vi "Channel Interface.vi"(8 "error in (no error)":errorcluster, 11 "Node Ptr":T1 format="%.0x") -> (0 "error out":errorcluster)   [LabVIEW 2017, in "SLSC EDS System Explorer.lvlib"]
uses:
  SLSC EDS System Explorer.lvlib
  <vilib>/NI Veristand/Custom Device API/Custom Device Item Ref.ctl
  <vilib>/NI Veristand/Custom Device API/Custom Device Channel Type.ctl
  <vilib>/NI Veristand/Custom Device Tools/Custom Device Utility Library/Search Direction.ctl
  <vilib>/Utility/miscctls.llb/LVStringsAndValuesArrayTypeDef_U16.ctl
  Shared/Constants.vi
  <vilib>/NI Veristand/Custom Device API/Get Item Property (String).vi
  <vilib>/NI Veristand/Custom Device Tools/Custom Device Utility Library/NI VeriStand - Search for Item by GUID.vi
  <vilib>/NI VeriStand/Custom Device API/Custom Device API.lvlib
  Shared/SLSC EDS Shared.lvlib
  <vilib>/NI VeriStand/Custom Device Tools/Custom Device Utility Library/Custom Device Utility Library.lvlib
  SLSC CD API/SLSC CD Shared/SLSC CD Shared.lvlib
  <vilib>/NI Veristand/Custom Device Tools/Custom Device Utility Library/NI VeriStand - Search for Item by Name.vi
  SLSC UI API/SLSC Tree Control.lvlib
  SLSC CD API/SLSC CD System Explorer/SLSC CD System Explorer.lvlib
panel:
  in  "Property tree":string[](tree)
  out "Physical Channel":string
  out "Property/Command Name":string
  out "Datatype":string
  in  "U8":u8 format="%.0x"
  in  "I8":i8
  in  "U32":u32 format="%.0x"
  in  "I32":i32
  in  "U64":u64 format="%.0x"
  in  "I64":i64
  in  "Ring":u16(ring)
  in  "DBL":dbl format="%#_16g"
  out "Documentation":string
  in  "Default Value":dbl
  out "Access":i32(ring) items=["None", "Read Only", "Write Only", "Read/Write"]
  out "SLSC Debugging Information":string
  in  "Header":cluster{"Section Name":string}={"Section Name"="Custom Device Item Settings"}
  out "Description":string
  out "Name":string
  # "Default Value"
  # "Channel Value"
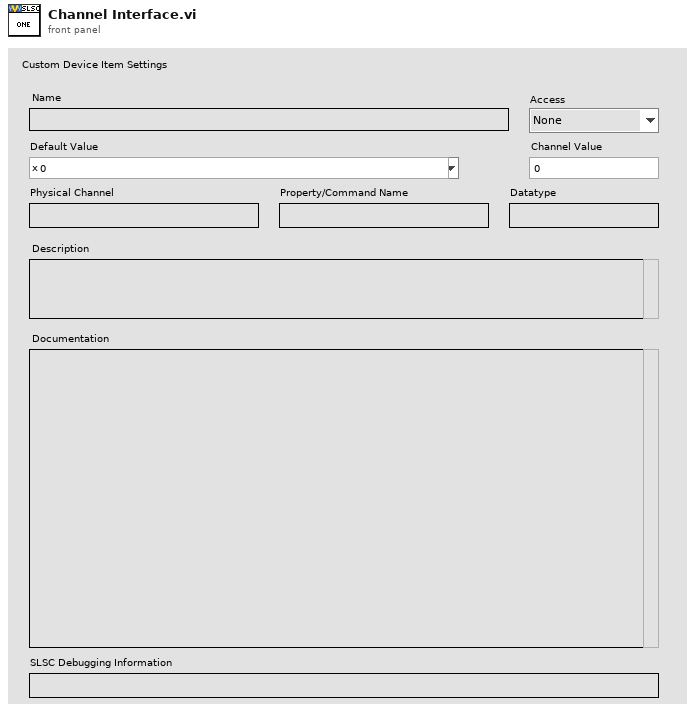
[diagram p1: front panel]
types:
  T1 = typedef "Custom Device API.lvlib/Custom Device Item Ref.ctl" = u64
  T2 = enum8{"Enabled", "Disabled", "Disabled and Grayed Out"}
  T3 = typedef "Custom Device Utility Library.lvlib/Search Direction.ctl" = enum16{"Down", "Up"}
  T4 = typedef "Custom Device API.lvlib/Custom Device Channel Type.ctl" = enum16{"Input", "Output"}
  T5 = typedef "LVStringsAndValuesArrayTypeDef_U16.ctl" = cluster{"String":string, "Value":u16}[]
  T6 = typedef "Custom Device API.lvlib/Custom Device Item Info.ctl" = cluster{"Name":string, "Is Channel":bool, "GUID":string, "Is Waveform":bool}
  T7 = typedef "EDSjsonStructure.ctl" = cluster{"vendorNum":u32, "vendorName":string, "vendorPrefix":string, "productNum":u32, "productName":string, "capsVersion":string, "capsSpecVersion":u32, "capsSpecOldestCompatibleVersion":u32, "enums":T8[], "properties":T9[], "commands":T10[], "scales":T11[], "physicalChannels":T12[], "registerMap":cluster{"registers":T13[]}}
  T8 = typedef "enum.ctl" = cluster{"name":string, "description-en":string, "values":cluster{"name":string, "description-en":string, "value":i32}[]}
  T9 = typedef "property.ctl" = cluster{"name":string, "description-en":string, "documentation-en":string, "dataType":string, "bitfield":string, "access":string, "scale":string, "value":variant, "min":variant, "max":variant, "default value":variant}
  T10 = typedef "command.ctl" = cluster{"name":string, "description-en":string, "documentation-en":string, "startBitfield":string, "waitTimeInMs":i32, "doneBitfield":string, "doneInterrupt":string, "doneTimeoutInMs":i32, "value":variant}
  T11 = typedef "scale.ctl" = cluster{"name":string, "description-en":string, "m":dbl, "b":dbl, "forwardCoeffs":dbl[], "reverseCoeffs":dbl[], "coercion":string, "table":cluster{"scaled":dbl, "unscaled":dbl}[]}
  T12 = typedef "physicalChannel.ctl" = cluster{"name":string, "description-en":string, "commands":T10[], "properties":T9[]}
  T13 = typedef "register.ctl" = cluster{"name":string, "description-en":string, "access":string, "address":u32, "size":u32, "bitfields":cluster{"name":string, "description-en":string, "offset":u32, "size":u32, "signed":bool, "strobe":bool}[]}
  T14 = typedef "Custom Device API.lvlib/Custom Device Channel.ctl" = cluster{"Type":T4, "Units":string, "Default Value":dbl, "Faultable":bool, "Scalable":bool}
  T15 = cluster{"Left Cell String":string, "Child Text":string[], "Child Tag":string, "Item Indent":i32, "Child Only?":bool, "Glyph Index":i32}[]
  T16 = cluster{"Left Cell String":string, "Child Text":string[], "Child Tag":string, "Item Indent":i32, "Child Only?":bool, "Glyph Index":i32}
  T17 = cluster{"name":string, "description-en":string, "value":i32}[]
  T18 = typedef "Custom Device API.lvlib/Custom Device Commands.ctl" = enum16{"Default", "Item renamed", "Shutdown", "Dynamic button pressed"}
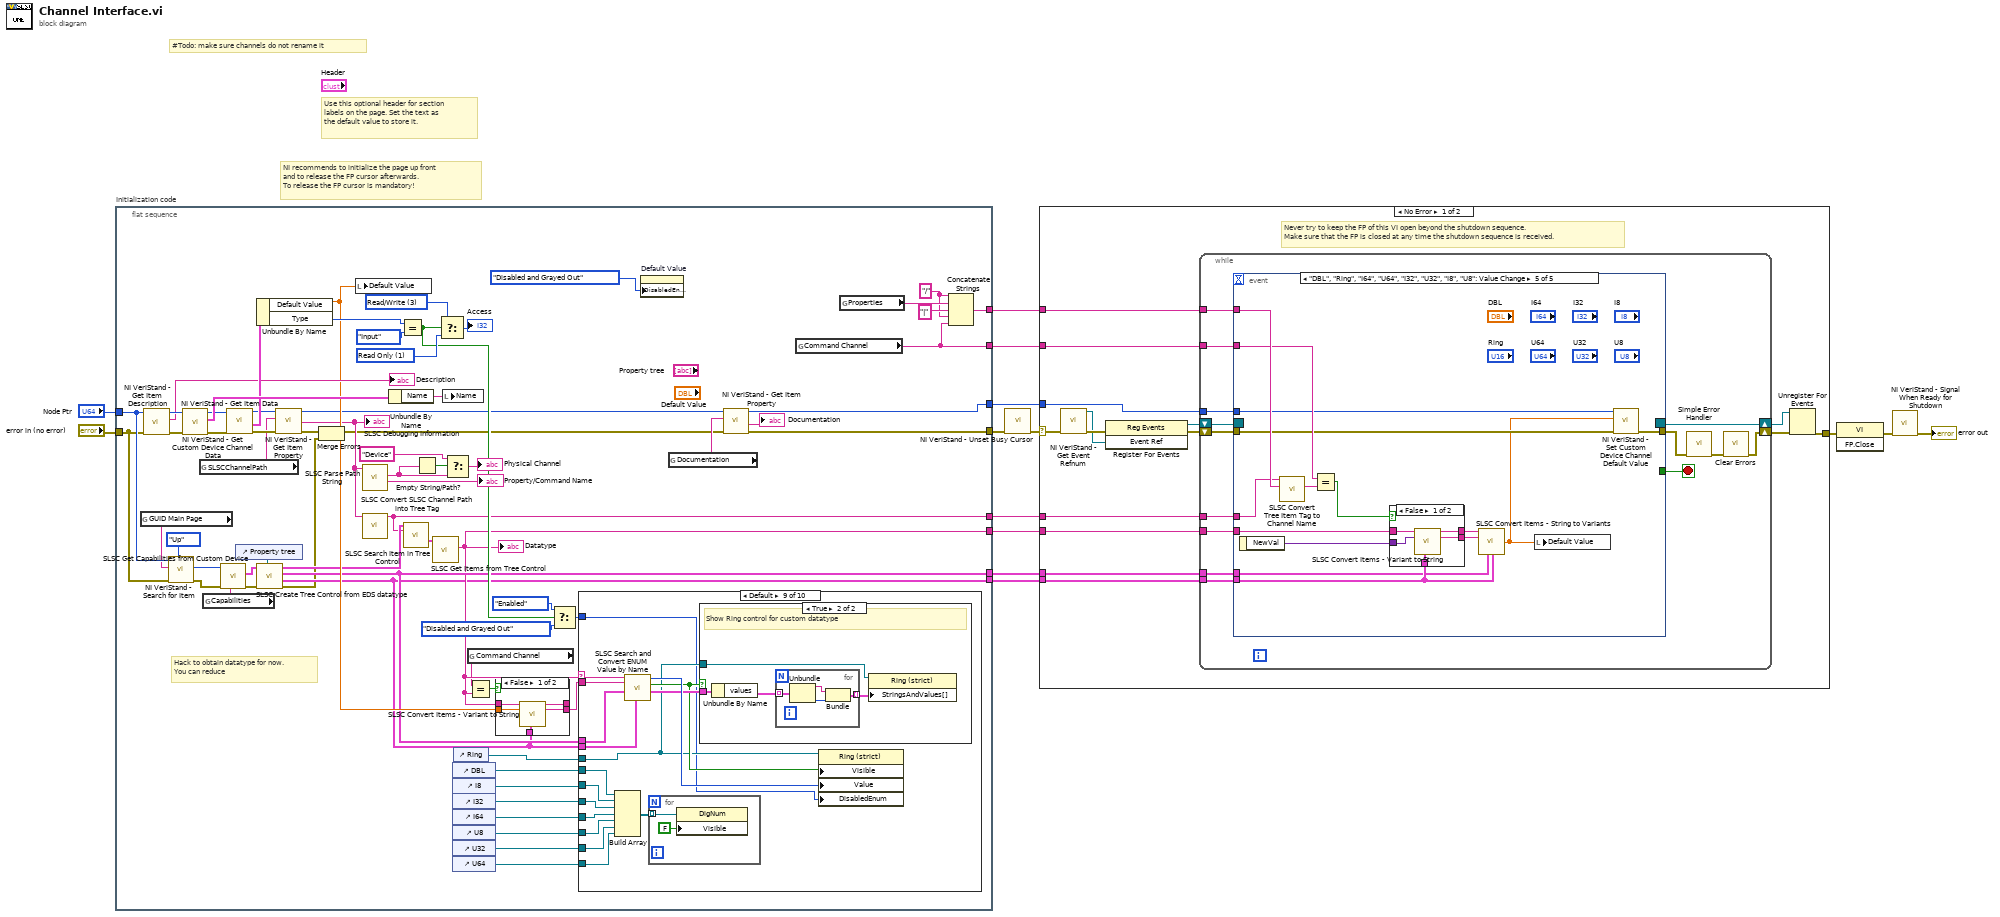
[diagram p0: block diagram]
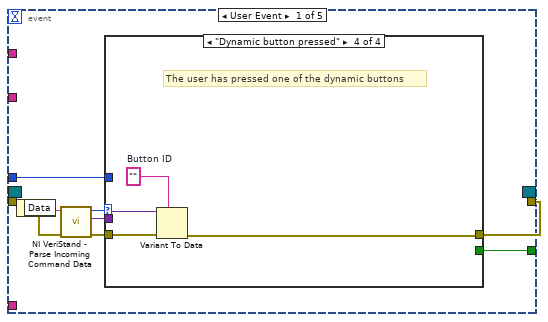
[diagram p2: hidden frame]
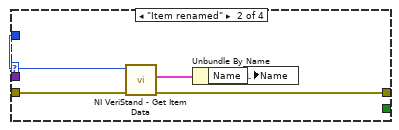
[diagram p4: hidden frame]
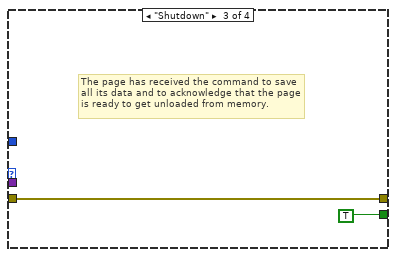
[diagram p5: hidden frame]
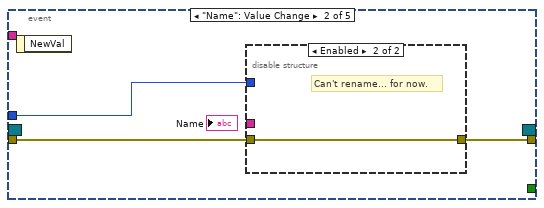
[diagram p6: hidden frame]
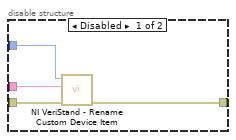
[diagram p7: hidden frame]
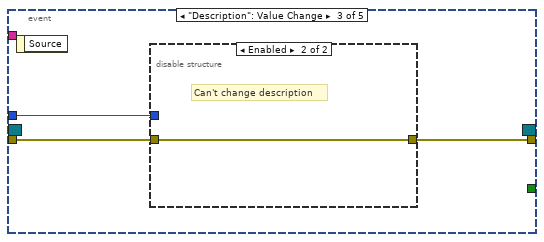
[diagram p8: hidden frame]
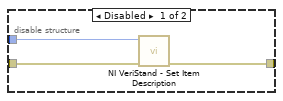
[diagram p9: hidden frame]
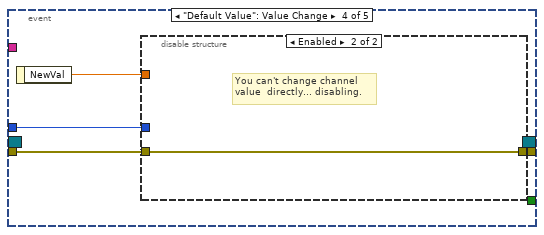
[diagram p10: hidden frame]
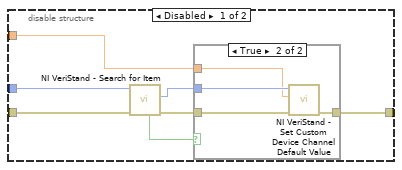
[diagram p11: hidden frame]
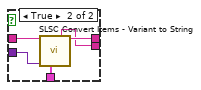
[diagram p13: hidden frame]
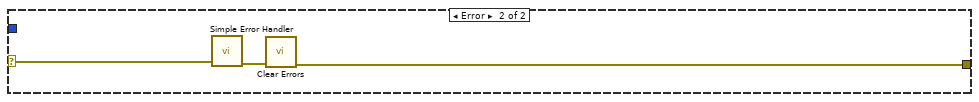
[diagram p14: hidden frame]
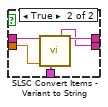
[diagram p15: hidden frame]
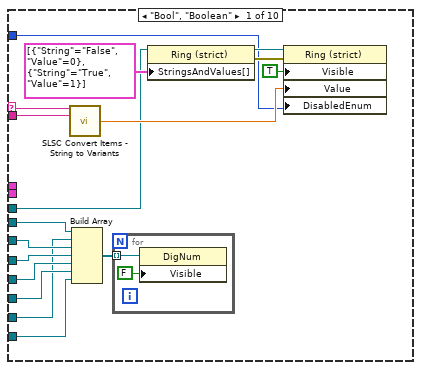
[diagram p16: hidden frame]
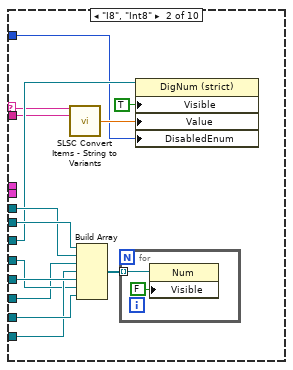
[diagram p17: hidden frame]
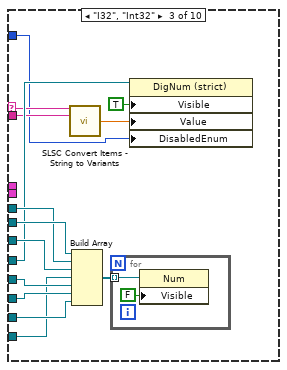
[diagram p18: hidden frame]
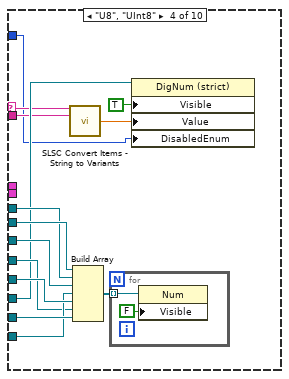
[diagram p19: hidden frame]
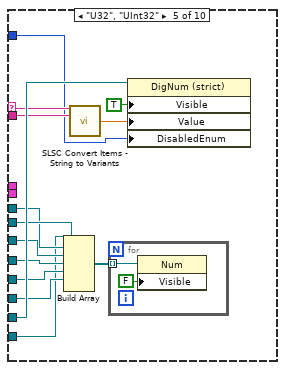
[diagram p20: hidden frame]
diagram:
  # "#Todo: make sure channels do not rename it"
  # "Use this optional header for section labels on the page. Set the text as the default value to store it."
  # "NI recommends to initialize the page up front\nand to release the FP cursor afterwards.\nTo release the FP cursor is mandatory!"
  n1 = flat-sequence "Initialization code" {
    tunnel: "error in (no error)" -> [w28]
    tunnel: "Node Ptr" -> [w53]
    tunnel: [w66] -> w10
    tunnel: [w23] -> w7
    tunnel: [w58] -> w6
    tunnel: [w49] -> w5
    tunnel: [w30] -> w4
    tunnel: [w36] -> w3
    tunnel: [w31] -> w2
    tunnel: [w32] -> w1
    frame #0 {
      w59 = "/" ("string")
      w79 = 1 items=["None", "Read Only", "Write Only", "Read/Write"] ("Access")
      w78 = 3 items=["None", "Read Only", "Write Only", "Read/Write"] ("Access")
      # "Hack to obtain datatype for now.\nYou can reduce"
      n2 = global read "Constants.vi" "GUID Main Page"() -> (w52:string)
      n3 = call <vilib>:"NI VeriStand - Get Item Description.vi"("error in (no error)"=w28, "Item Ref in"=w53) -> ("error out"=w81:errorcluster, "Description"=→"Description":string, "Item Ref out"=w82:T1)  [unwired: 7 out]
      n4 = call-poly <vilib>:"NI VeriStand - Search for Item.vi"("Direction (Down)"=Search_Direction."Up", "error in"=w28, "Item GUID"=w52, "Section Ref in"=w53) -> ("error out"=w29:errorcluster, "Item Ref"=w54:T1)  [unwired: 4 in, 2 out]
      n5 = call <vilib>:"NI VeriStand - Get Item Data.vi"("error in (no error)"=w81, "Item Ref in"=w82) -> ("error out"=w71:errorcluster, "Item Info"=w80:T6, "Item Ref out"=w72:T1)  [unwired: 7 out]
      n6 = global read "Constants.vi" "SLSCChannelPath"() -> (w70:string)
      n7 = global read "Constants.vi" "Capabilities"() -> (w62:string)
      n8 = call "SLSC Get Capabilities from Custom Device.vi"("Property Name"=w62, "error in (no error)"=w29, "Device Item Ref in"=w54) -> ("error out"=w25:errorcluster, "data"=w37:T7)  [unwired: 3 in, 4 out]
      n9 = call <vilib>:"NI VeriStand - Get Custom Device Channel Data.vi"("error in (no error)"=w71, "Channel Ref in"=w72) -> ("error out"=w74:errorcluster, "Channel"=w73:T14, "Channel Ref out"=w68:T1)  [unwired: 4 in, 3 out]
      n10 = control-ref of="Property tree"() -> (w38:refnum<vi>)
      n11 = Unbundle By Name(w73) -> ("Default Value"=w50:dbl, "Type"=w75:T4)
      n12 = call "SLSC Create Tree Control from EDS datatype.vi"("Property Tree"=w38, "error in (no error)"=w25, "SLSC EDS module"=w37) -> ("error out"=w19:errorcluster, "Enum Strings"=w30:cluster{"name":string, string}[], "Enums"=w36:T8[], "SLSC Output Tree"=w35:T15)  [unwired: 5 in]
      n13 = call-poly <vilib>:"NI VeriStand - Get Item Property.vi"("error in (no error)"=w74, "Property Name"=w70, "Item Ref in"=w68) -> ("error out"=w21:errorcluster, "Value"=w34:string, "Item Ref out"=w22:T1)  [unwired: 5 in, 1 out]
      "SLSC Debugging Information" <- w34
      n14 = Merge Errors(w21, w19) -> (w20:errorcluster)
      n15 = local write "Default Value"(w50) -> ()
      n16 = call "SLSC Parse Path String.vi"("SLSC Channel Path"=w34) -> ("Property or Command"=→"Property/Command Name":string, "Physical Channel"=w40:string)  [unwired: 7 in, 2 out]
      n17 = call "SLSC Convert SLSC Channel Path into Tree Tag.vi"("SLSC Channel Path"=w34) -> ("Tree Item Channel"=w32:string)  [unwired: 9 in, 1 out]
      n18 = Unbundle By Name(w80) -> ("Name"=w63:string)
      n19 = Equal?(x=w75, y=Custom_Device_Channel_Type."Input") -> (x = y?=w64:bool)
      n20 = call "SLSC Search Item in Tree Control.vi"("SLSC Output Tree"=w35, "Item Tag"=w32) -> ("Item"=w33:T16)  [unwired: 10 in, 3 out]
      n21 = Empty String/Path?(string/path=w40) -> (empty?=w42:bool)
      n22 = call "SLSC Get Items from Tree Control.vi"("Item"=w33) -> ("Datatype"=w31:string)  [unwired: 6 in, 4 out]
      "Datatype" <- w31
      n23 = Select(t=w78, s=w64, f=w79) -> (s? t:f=→"Access":i32)
      n24 = local write "Name"(w63) -> ()
      n25 = Select(t="Device", s=w42, f=w40) -> (s? t:f=→"Physical Channel":string)
      n26 = control-ref of="DBL"() -> (w44:refnum<vi>)
      n27 = control-ref of="I8"() -> (w57:refnum<vi>)
      n28 = control-ref of="I32"() -> (w56:refnum<vi>)
      n29 = control-ref of="I64"() -> (w45:refnum<vi>)
      n30 = control-ref of="U8"() -> (w48:refnum<vi>)
      n31 = control-ref of="U32"() -> (w47:refnum<vi>)
      n32 = control-ref of="U64"() -> (w46:refnum<vi>)
      n33 = control-ref of="Ring"() -> (w16:refnum<vi>)
      n34 = global read "Constants.vi" "Command Channel"() -> (w24:string)
      n35 = Equal?(x=w24, y=w31) -> (x = y?=w27:bool)
      n36 = case shown="False" w27 {
        tunnel: w50 -> [w87 w89]
        tunnel: [w86 w88] -> w26
        tunnel: [w85 w92] -> _
        tunnel: w31 -> [w84 w91]
        tunnel: w30 -> [w83 w90]
        frame False {
          n37 = call "SLSC Convert Items - Variant to String.vi"("Datatype"=w84, "value"=w87, "Enum string"=w83) -> ("Output data type"=w85:string, "string data value"=w86:string)  [unwired: 6 in, 5 out]
        }
        frame True {
          n38 = call "SLSC Convert Items - Variant to String.vi"("Datatype"=w91, "reset value"=w89, "Enum string"=w90) -> ("string data reset value"=w88:string, "Output data type"=w92:string)  [unwired: 6 in, 5 out]
        }
      }
      n39 = Select(t=T2."Enabled" ("Disabled"), s=w64, f=T2."Disabled and Grayed Out" ("Disabled")) -> (s? t:f=w15:T2)
      n40 = case shown="Default" w31 {
        selector: w31 -> [w99 w116 w132 w148 w164 w178 w198 w216 w233 w264]
        tunnel: w16 -> [w95 w124 w140 w156 w171 w190 w208 w225 w229 w256]
        tunnel: w47 -> [w102 w121 w135 w152 w173 w185 w202 w219 w238 w268]
        tunnel: w44 -> [w109 w125 w141 w157 w172 w191 w209 w218 w243 w273]
        tunnel: w57 -> [w108 w117 w139 w155 w170 w189 w207 w224 w242 w272]
        tunnel: w56 -> [w107 w119 w133 w150 w169 w188 w206 w223 w241 w271]
        tunnel: w45 -> [w106 w123 w138 w154 w168 w183 w205 w222 w240 w270]
        tunnel: w48 -> [w105 w118 w137 w149 w167 w187 w204 w221 w239 w269]
        tunnel: w46 -> [w104 w120 w134 w151 w166 w184 w201 w217 w237 w267]
        tunnel: w36 -> [_ _ _ _ _ _ _ _ w244 _]
        tunnel: w26 -> [w98 w115 w131 w147 w163 w177 w197 w215 w235 w265]
        tunnel: w30 -> [_ _ _ _ _ _ _ _ w234 _]
        tunnel: w15 -> [w93 w112 w128 w144 w160 w176 w194 w212 w228 _]
        frame "Bool", "Boolean" {
          n41 = call "SLSC Convert Items - String to Variants.vi"("Datatype"=w99, "Value"=w98) -> ("Value (DBL)"=w97:dbl)  [unwired: 10 in, 3 out]
          n42 = Build Array(w109, w102, w108, w107, w106, w105, w104) -> (w103:refnum<vi>[])
          n43 = for {
            tunnel: w103 -> [w111] mode=indexing
            n44 = property class="DigNum"(reference=w111, "Visible"=FALSE) -> ()  [unwired: 1 in, 2 out]
          }
          n45 = property on="Property Node" class="Ring (strict)"(reference=w95, "StringsAndValues[]"=T5 [{"String"="False", "Value"=0}, {"String"="True", "Value"=1}] ("Strings And Values []")) -> (reference out=w94:refnum<vi>, error out=w100:errorcluster)  [unwired: 1 in]
          n46 = property class="Ring (strict)"(reference=w94, error in=w100, "Visible"=TRUE, "Value"=w97, "DisabledEnum"=w93) -> ()  [unwired: 2 out]
        }
        frame "I8", "Int8" {
          n47 = call "SLSC Convert Items - String to Variants.vi"("Datatype"=w116, "Value"=w115) -> ("Value (DBL)"=w114:dbl)  [unwired: 10 in, 3 out]
          n48 = Build Array(w125, w124, w118, w120, w123, w119, w121) -> (w122:refnum<vi>[])
          n49 = for {
            tunnel: w122 -> [w127] mode=indexing
            n50 = property class="Num"(reference=w127, "Visible"=FALSE) -> ()  [unwired: 1 in, 2 out]
          }
          n51 = property class="DigNum (strict)"(reference=w117, "Visible"=TRUE, "Value"=w114, "DisabledEnum"=w112) -> ()  [unwired: 1 in, 2 out]
        }
        frame "I32", "Int32" {
          n52 = call "SLSC Convert Items - String to Variants.vi"("Datatype"=w132, "Value"=w131) -> ("Value (DBL)"=w130:dbl)  [unwired: 10 in, 3 out]
          n53 = Build Array(w141, w140, w139, w134, w138, w137, w135) -> (w136:refnum<vi>[])
          n54 = for {
            tunnel: w136 -> [w143] mode=indexing
            n55 = property class="Num"(reference=w143, "Visible"=FALSE) -> ()  [unwired: 1 in, 2 out]
          }
          n56 = property class="DigNum (strict)"(reference=w133, "Visible"=TRUE, "Value"=w130, "DisabledEnum"=w128) -> ()  [unwired: 1 in, 2 out]
        }
        frame "U8", "UInt8" {
          n57 = call "SLSC Convert Items - String to Variants.vi"("Datatype"=w148, "Value"=w147) -> ("Value (DBL)"=w146:dbl)  [unwired: 10 in, 3 out]
          n58 = Build Array(w157, w156, w155, w151, w154, w150, w152) -> (w153:refnum<vi>[])
          n59 = for {
            tunnel: w153 -> [w159] mode=indexing
            n60 = property class="Num"(reference=w159, "Visible"=FALSE) -> ()  [unwired: 1 in, 2 out]
          }
          n61 = property class="DigNum (strict)"(reference=w149, "Visible"=TRUE, "Value"=w146, "DisabledEnum"=w144) -> ()  [unwired: 1 in, 2 out]
        }
        frame "U32", "UInt32" {
          n62 = Build Array(w172, w171, w170, w169, w168, w167, w166) -> (w165:refnum<vi>[])
          n63 = call "SLSC Convert Items - String to Variants.vi"("Datatype"=w164, "Value"=w163) -> ("Value (DBL)"=w162:dbl)  [unwired: 10 in, 3 out]
          n64 = for {
            tunnel: w165 -> [w175] mode=indexing
            n65 = property class="Num"(reference=w175, "Visible"=FALSE) -> ()  [unwired: 1 in, 2 out]
          }
          n66 = property class="DigNum (strict)"(reference=w173, "Visible"=TRUE, "Value"=w162, "DisabledEnum"=w160) -> ()  [unwired: 1 in, 2 out]
        }
        frame "I64", "Int64" {
          n67 = call "SLSC Convert Items - String to Variants.vi"("Datatype"=w178, "Value"=w177) -> ("Value"=w182:variant)  [unwired: 10 in, 3 out]
          n68 = Build Array(w191, w190, w189, w188, w184, w187, w185) -> (w186:refnum<vi>[])
          n69 = for {
            tunnel: w186 -> [w193] mode=indexing
            n70 = property class="Num"(reference=w193, "Visible"=FALSE) -> ()  [unwired: 1 in, 2 out]
          }
          n71 = Variant To Data(type=i64 0, Variant=w182) -> (data=w180:i64)  [unwired: 1 in, 1 out]
          n72 = property class="DigNum (strict)"(reference=w183, "Visible"=TRUE, "Value"=w180, "DisabledEnum"=w176) -> ()  [unwired: 1 in, 2 out]
        }
        frame "U64", "UInt64" {
          n73 = call "SLSC Convert Items - String to Variants.vi"("Datatype"=w198, "Value"=w197) -> ("Value"=w196:variant)  [unwired: 10 in, 3 out]
          n74 = Build Array(w209, w208, w207, w206, w205, w204, w202) -> (w203:refnum<vi>[])
          n75 = for {
            tunnel: w203 -> [w211] mode=indexing
            n76 = property class="Num"(reference=w211, "Visible"=FALSE) -> ()  [unwired: 1 in, 2 out]
          }
          n77 = Variant To Data(type=u64 0, Variant=w196) -> (data=w199:u64)  [unwired: 1 in, 1 out]
          n78 = property class="DigNum (strict)"(reference=w201, "Visible"=TRUE, "Value"=w199, "DisabledEnum"=w194) -> ()  [unwired: 1 in, 2 out]
        }
        frame "DBL", "Double" {
          n79 = call "SLSC Convert Items - String to Variants.vi"("Datatype"=w216, "Value"=w215) -> ("Value (DBL)"=w214:dbl)  [unwired: 10 in, 3 out]
          n80 = Build Array(w217, w225, w224, w223, w222, w221, w219) -> (w220:refnum<vi>[])
          n81 = for {
            tunnel: w220 -> [w227] mode=indexing
            n82 = property class="Num"(reference=w227, "Visible"=FALSE) -> ()  [unwired: 1 in, 2 out]
          }
          n83 = property class="DigNum (strict)"(reference=w218, "Visible"=TRUE, "Value"=w214, "DisabledEnum"=w212) -> ()  [unwired: 1 in, 2 out]
        }
        frame Default {
          n84 = Build Array(w243, w242, w241, w240, w239, w238, w237) -> (w236:refnum<vi>[])
          n85 = call "SLSC Search and Convert ENUM Value by Name.vi"("Enum Strings"=w234, "enums"=w244, "Value"=w235, "Datatype Name"=w233) -> ("Enum"=w231:T8, "Datatype found?"=w230:bool, "Value"=w232:i32)  [unwired: 5 in]
          n86 = for {
            tunnel: w236 -> [w246] mode=indexing
            n87 = property class="DigNum"(reference=w246, "Visible"=FALSE) -> ()  [unwired: 1 in, 2 out]
          }
          n88 = case shown="True" w230 {
            tunnel: w231 -> [_ w250]
            tunnel: w229 -> [_ w247]
            frame False {
              # "Datatype not found: hide all controls"
            }
            frame True {
              # "Show Ring control for custom datatype"
              n89 = Unbundle By Name(w250) -> ("values"=w249:T17)
              n90 = for {
                tunnel: w249 -> [w254] mode=indexing
                tunnel: [w251] -> w248 mode=indexing
                n91 = Unbundle(w254) -> ("name"=w253:string, "value"=w252:i32)  [unwired: 1 out]
                n92 = Bundle("name"=w253, "value"=w252) -> (w251:cluster{"name":string, "value":i32})  [unwired: 1 in]
              }
              n93 = property on="Property Node" class="Ring (strict)"(reference=w247, "StringsAndValues[]"=w248) -> ()  [unwired: 1 in, 2 out]
            }
          }
          n94 = property class="Ring (strict)"(reference=w229, "Visible"=w230, "Value"=w232, "DisabledEnum"=w228) -> ()  [unwired: 1 in, 2 out]
        }
        frame "Command" {
          n95 = Build Array(w273, w272, w271, w270, w269, w268, w267) -> (w266:refnum<vi>[])
          n96 = call "SLSC Command Enum Constant.vi"("Option on Reset?"=FALSE) -> ("Array"=w261:T8[])  [unwired: 10 in, 4 out]
          n97 = for {
            tunnel: w266 -> [w279] mode=indexing
            n98 = property class="DigNum"(reference=w279, "Visible"=FALSE) -> ()  [unwired: 1 in, 2 out]
          }
          n99 = call "SLSC Search and Convert ENUM Value by Name.vi"("enums"=w261, "Value"=w265, "Datatype Name"=w264) -> ("Enum"=w262:T8, "Value"=w263:i32)  [unwired: 6 in, 1 out]
          n100 = Unbundle By Name(w262) -> ("values"=w259:T17)
          n101 = for {
            tunnel: w259 -> [w277] mode=indexing
            tunnel: [w274] -> w258 mode=indexing
            n102 = Unbundle(w277) -> ("name"=w276:string, "value"=w275:i32)  [unwired: 1 out]
            n103 = Bundle("name"=w276, "value"=w275) -> (w274:cluster{"name":string, "value":i32})  [unwired: 1 in]
          }
          n104 = property class="Ring (strict)"(reference=w256, "Visible"=TRUE, "Value"=w263, "DisabledEnum"=T2."Disabled and Grayed Out" ("Disabled")) -> ()  [unwired: 1 in, 2 out]
          n105 = property on="Property Node" class="Ring (strict)"(reference=w256, "StringsAndValues[]"=w258) -> ()  [unwired: 1 in, 2 out]
        }
      }
      n106 = property on="Default Value" class="DigNum (strict)"("DisabledEnum"=T2."Disabled and Grayed Out" ("Disabled")) -> ()  [unwired: 2 in, 2 out]
      n107 = global read "Constants.vi" "Documentation"() -> (w69:string)
      n108 = call-poly <vilib>:"NI VeriStand - Get Item Property.vi"("error in (no error)"=w20, "Property Name"=w69, "Item Ref in"=w22) -> ("error out"=w66:errorcluster, "Value"=→"Documentation":string, "Item Ref out"=w23:T1)  [unwired: 5 in, 1 out]
      n109 = global read "Constants.vi" "Command Channel"() -> (w49:string)
      n110 = global read "Constants.vi" "Properties"() -> (w60:string)
      n111 = Concatenate Strings(w59, w60, "|" ("string"), w59, w49) -> (w58:string)
    }
  }
  n112 = call <vilib>:"NI VeriStand - Unset Busy Cursor.vi"("error in (no error)"=w10) -> ("error out"=w9:errorcluster)  [unwired: 10 out]
  n113 = case shown="No Error" w9 {
    selector: w9 -> [w286 w386]
    tunnel: [w291 w387] -> w14
    tunnel: w7 -> [w287 _]
    tunnel: w1 -> [w285 _]
    tunnel: w6 -> [w284 _]
    tunnel: w5 -> [w283 _]
    tunnel: w4 -> [w282 _]
    tunnel: w3 -> [w281 _]
    tunnel: w2 -> [w280 _]
    frame No Error {
      # "Never try to keep the FP of this VI open beyond the shutdown sequence.\nMake sure that the FP is closed at any time the shutdown sequence is received."
      n114 = call <vilib>:"NI VeriStand - Get Event Refnum.vi"("error in (no error)"=w286) -> ("error out"=w294:errorcluster, "Event Ref"=w290:refnum<user-event>)  [unwired: 9 out]
      n115 = register-events(error in=w294, w290) -> (reference out=w288:refnum<event-registration>, error out=w289:errorcluster)  [unwired: 1 in]
      n116 = while {
        tunnel: w287 -> [w304]
        shift-right: [w302] -> w292
        shift-left: w289 -> [w307]
        shift-right: [w308] -> w293
        shift-left: w288 -> [w306]
        tunnel: w285 -> [w301]
        tunnel: w284 -> [w300]
        tunnel: w283 -> [w299]
        tunnel: w282 -> [w298]
        tunnel: w281 -> [w297]
        tunnel: w280 -> [w296]
        stop <- w305 stop-if-true
        n117 = event shown="[4] \"DBL\", \"Ring\", \"I64\", \"U64\", \"I32\", \"U32\", \"I8\", \"U8\": Value Change" {
          selector: w306 -> [_ _ _ _ _]
          dyn-events: [_ _ _ _ _] -> w308
          timeout: _ -> [_ _ _ _ _]
          tunnel: w307 -> [w316 w331 w338 w345 w366]
          tunnel: [w312 _ _ _ _] -> w305
          tunnel: [w311 w330 w337 w344 w368] -> w295
          tunnel: w304 -> [w310 w329 w339 w347 w367]
          tunnel: w301 -> [_ _ _ _ w361]
          tunnel: w300 -> [_ _ _ _ w371]
          tunnel: w299 -> [_ _ _ _ w370]
          tunnel: w298 -> [_ _ _ _ w364]
          tunnel: w297 -> [_ _ _ _ w363]
          tunnel: w296 -> [_ _ _ _ w362]
          event User Event {
            n118 = event-data() -> ("Data"=w315:string)  [unwired: 1 out]
            n119 = call <vilib>:"NI VeriStand - Parse Incoming Command Data.vi"("error in (no error)"=w316, "Incoming data"=w315) -> ("error out"=w314:errorcluster, "Outgoing data"=w309:variant, "Action"=w313:T18)  [unwired: 7 out]
            n120 = case shown="\"Dynamic button pressed\"" w313 {
              tunnel: w314 -> [w317 w322 w323 w328]
              tunnel: [_ _ TRUE _] -> w312
              tunnel: [w317 w319 w323 w325] -> w311
              tunnel: w310 -> [_ w321 _ _]
              tunnel: w309 -> [_ _ _ w327]
              frame "Default", Default {
              }
              frame "Item renamed" {
                n121 = call <vilib>:"NI VeriStand - Get Item Data.vi"("error in (no error)"=w322, "Item Ref in"=w321) -> ("error out"=w319:errorcluster, "Item Info"=w320:T6)  [unwired: 8 out]
                n122 = Unbundle By Name(w320) -> ("Name"=w318:string)
                n123 = local write "Name"(w318) -> ()
              }
              frame "Shutdown" {
                # "The page has received the command to save all its data and to acknowledge that the page is ready to get unloaded from memory."
              }
              frame "Dynamic button pressed" {
                w326 = ""  # Button ID
                # "The user has pressed one of the dynamic buttons"
                n124 = Variant To Data(error in=w328, type=w326, Variant=w327) -> (error out=w325:errorcluster)  [unwired: 1 out]
              }
            }
          }
          event "Name": Value Change {
            n125 = event-data() -> ()  [unwired: 2 out]
            n126 = disable-structure shown="Enabled" {
              disable-tunnel: w331 -> [w335 w336]
              disable-tunnel: [w334 w336] -> w330
              disable-tunnel: w329 -> [w333 _]
              disable-tunnel: _ -> [w332 _]
              frame Disabled {
                n127 = call <vilib>:"NI VeriStand - Rename Custom Device Item.vi"("error in (no error)"=w335, "New Name"=w332, "Item Ref in"=w333) -> ("error out"=w334:errorcluster)  [unwired: 1 in, 7 out]
              }
              frame Enabled {
                # "Can't rename... for now."
              }
            }
          }
          event "Description": Value Change {
            n128 = event-data() -> ()  [unwired: 2 out]
            n129 = disable-structure shown="Enabled" {
              disable-tunnel: w339 -> [w342 _]
              disable-tunnel: w338 -> [w341 w343]
              disable-tunnel: [w340 w343] -> w337
              frame Disabled {
                n130 = call <vilib>:"NI VeriStand - Set Item Description.vi"("error in (no error)"=w341, "Item Ref in"=w342) -> ("error out"=w340:errorcluster)  [unwired: 1 in, 8 out]
              }
              frame Enabled {
                # "Can't change description"
              }
            }
          }
          event "Default Value": Value Change {
            n131 = event-data() -> ("NewVal"=w346:dbl)  [unwired: 1 out]
            n132 = disable-structure shown="Enabled" {
              disable-tunnel: w347 -> [w354 _]
              disable-tunnel: w346 -> [w352 _]
              disable-tunnel: w345 -> [w351 w360]
              disable-tunnel: [w349 w360] -> w344
              frame Disabled {
                n133 = call-poly <vilib>:"NI VeriStand - Search for Item.vi"("error in"=w351, "Section Ref in"=w354) -> ("error out"=w350:errorcluster, "Item Ref"=w353:T1, "Found"=w348:bool)  [unwired: 6 in, 1 out]
                n134 = case shown="True" w348 {
                  tunnel: w353 -> [_ w359]
                  tunnel: w352 -> [_ w358]
                  tunnel: w350 -> [w355 w357]
                  tunnel: [w355 w356] -> w349
                  frame False {
                  }
                  frame True {
                    n135 = call <vilib>:"NI VeriStand - Set Custom Device Channel Default Value.vi"("error in (no error)"=w357, "Default Value"=w358, "Channel Ref in"=w359) -> ("error out"=w356:errorcluster)  [unwired: 7 in, 1 out]
                  }
                }
              }
              frame Enabled {
                # "You can't change channel \nvalue  directly... disabling."
              }
            }
          }
          event "DBL", "Ring", "I64", "U64", "I32", "U32", "I8", "U8": Value Change {
            n136 = event-data() -> ("NewVal"=w375:variant)  [unwired: 1 out]
            n137 = call "SLSC Convert Tree Item Tag to Channel Name.vi"("Type of Item"=w371, "Item String"=w361) -> ("Type of Item"=w372:string)  [unwired: 7 in, 2 out]
            n138 = Equal?(x=w370, y=w372) -> (x = y?=w369:bool)
            n139 = case shown="False" w369 {
              tunnel: w375 -> [w380 w382]
              tunnel: [w379 w381] -> w373
              tunnel: [w378 w385] -> w374
              tunnel: w362 -> [w377 w384]
              tunnel: w364 -> [w376 w383]
              frame False {
                n140 = call "SLSC Convert Items - Variant to String.vi"("Datatype"=w377, "value"=w380, "Enum string"=w376) -> ("Output data type"=w378:string, "string data value"=w379:string)  [unwired: 6 in, 5 out]
              }
              frame True {
                n141 = call "SLSC Convert Items - Variant to String.vi"("Datatype"=w384, "reset value"=w382, "Enum string"=w383) -> ("string data reset value"=w381:string, "Output data type"=w385:string)  [unwired: 6 in, 5 out]
              }
            }
            n142 = call "SLSC Convert Items - String to Variants.vi"("Datatype"=w374, "Value"=w373, "enums"=w363, "string enums"=w364) -> ("Value (DBL)"=w365:dbl)  [unwired: 8 in, 3 out]
            n143 = local write "Default Value"(w365) -> ()
            n144 = call <vilib>:"NI VeriStand - Set Custom Device Channel Default Value.vi"("error in (no error)"=w366, "Default Value"=w365, "Channel Ref in"=w367) -> ("error out"=w368:errorcluster)  [unwired: 7 in, 1 out]
          }
        }
        n145 = call <vilib>:"Simple Error Handler.vi"("error in (no error)"=w295) -> ("error out"=w303:errorcluster)  [unwired: 1 in, 7 out]
        n146 = call <vilib>:"Clear Errors.vi"("error in (no error)"=w303) -> ("error out"=w302:errorcluster)  [unwired: 1 in, 5 out]
      }
      n147 = Unregister For Events(event registration refnum=w293, error in=w292) -> (error out=w291:errorcluster)
    }
    frame Error {
      n148 = call <vilib>:"Simple Error Handler.vi"("error in (no error)"=w386) -> ("error out"=w388:errorcluster)  [unwired: 1 in, 7 out]
      n149 = call <vilib>:"Clear Errors.vi"("error in (no error)"=w388) -> ("error out"=w387:errorcluster)  [unwired: 1 in, 5 out]
    }
  }
  n150 = invoke class="VI" method="FP.Close"(error in=w14) -> (error out=w13:errorcluster)  [unwired: 2 in, 2 out]
  n151 = call <vilib>:"NI VeriStand - Signal When Ready for Shutdown.vi"("error in (no error)"=w13) -> ("error out"=→"error out":errorcluster)  [unwired: 10 out]
